vi "Prefilter_LP.vi"(8 "error in (no error)":errorcluster, 10 "low cutoff freq [Hz]":dbl=0.45, 11 "Waveforms In":waveform(dbl)[](array[waveform])) -> (0 "error out":errorcluster, 3 "Waveforms Out":waveform(dbl)[](array[waveform]))   [LabVIEW 2020, in "DSP_Filter.lvclass"]
uses:
  DSP_Filter.lvclass
  <vilib>/addons/Digital Filter Design/Process.llb/DFD Filtering (Wfm NChan).vi
  <vilib>/addons/Digital Filter Design/NI_DigFilterLicensed.lvlib
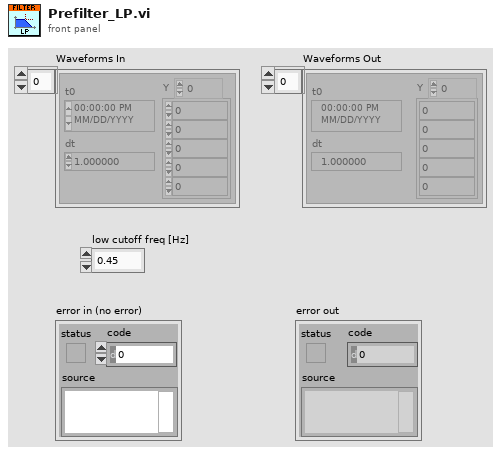
[diagram p1: front panel]
types:
  T1 = enum16{"Lowpass", "Highpass", "Bandpass", "Bandstop"}
  T2 = typedef "NI_DigFilterLicensed.lvlib/DFD Filter Obj.ctl" = cluster{"mSRate_Fs":dbl, "mSRate_Version":string, "mSRate_Comments":string, "mSRate_OrgCoef":T3, "mSRate_CurCoef":T3, "mSRate_Quantized?":bool, "mSRate_QCoef":T3, "mSRate_QSettings":T5[], "mSRate_Order":i32, "mSRate_Scaling":cluster{"mSRate_ScaleByPowerOf2?":bool, "mSRate_ScaleType":T7}}
  T3 = typedef "NI_DigFilterLicensed.lvlib/DFD Filter Coef.ctl" = cluster{"type":T4, "gain":dbl, "coef a (k)":dbl[], "coef b (v)":dbl[]}
  T4 = typedef "NI_DigFilterLicensed.lvlib/DFD Filter Structure Type Selector.ctl" = enum16{"Undefined", "FIR Direct Form", "FIR Direct Form Transposed", "FIR Symmetric", "FIR Antisymmetric", "IIR Direct Form I", "IIR Direct Form I Transposed", "IIR Direct Form II", "IIR Direct Form II Transposed", "IIR Cascaded Second Order Sections Form I", "IIR Cascaded Second Order Sections Form I Transposed", "IIR Cascaded Second Order Sections Form II", "IIR Cascaded Second Order Sections Form II Transposed", "Lattice Allpass (basic sections)", "Lattice Allpass (one multiplier sections)", "Lattice Allpass (normalized sections)", "Lattice AR (basic sections)", "Lattice AR (one multiplier sections)", "Lattice AR (normalized sections)", "Lattice MA (minimum phase)", "Lattice MA (maximum phase)", "Lattice ARMA (basic sections)", "Lattice ARMA (one multiplier sections)", "Lattice ARMA (normalized sections)"}
  T5 = typedef "NI_DigFilterLicensed.lvlib/dfd_Internal Quantization Settings.ctl" = cluster{"source":T6, "wl":i16, "iwl":i16, "overflow mode":enum16{"Saturation", "Wrap"}, "rounding mode":enum16{"Nearest", "Truncation"}, "signed?":bool}
  T6 = typedef "NI_DigFilterLicensed.lvlib/dfd_Internal Quantization Srcs.ctl" = u16
  T7 = typedef "NI_DigFilterLicensed.lvlib/DFD Coef Norm Type.ctl" = enum16{"No Norm", "Time Domain 1-Norm", "Time Domain 2-Norm", "Time Domain Inf-Norm"}
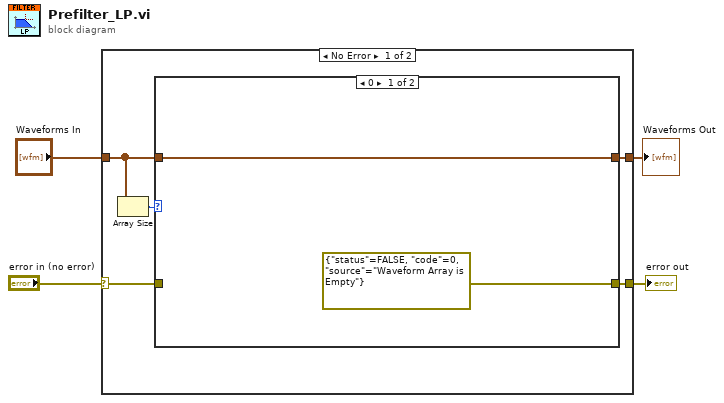
[diagram p0: block diagram]
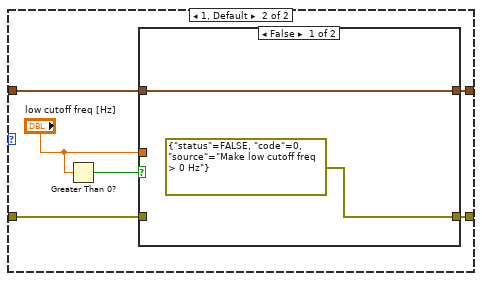
[diagram p2: hidden frame]
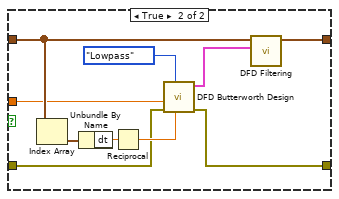
[diagram p3: hidden frame]
diagram:
  n1 = case shown="No Error" "error in (no error)" {
    selector: "error in (no error)" -> [w7 w30]
    tunnel: "Waveforms In" -> [w5 w31]
    tunnel: [w9 w31] -> w3
    tunnel: [w8 w30] -> w2
    frame No Error {
      n2 = Array Size(array=w5) -> (size(s)=w6:i32)
      n3 = case shown="0" w6 {
        tunnel: w5 -> [w10 w17]
        tunnel: [w10 w16] -> w9
        tunnel: [errorcluster {"status"=FALSE, "code"=0, "source"="Waveform Array is Empty"} ("error constant") w15] -> w8
        tunnel: w7 -> [_ w14]
        frame 0 {
        }
        frame 1, Default {
          n4 = Greater Than 0?(x="low cutoff freq [Hz]") -> (x > 0?=w12:bool)
          n5 = case shown="False" w12 {
            tunnel: w17 -> [w19 w27]
            tunnel: [w19 w26] -> w16
            tunnel: [errorcluster {"status"=FALSE, "code"=0, "source"="Make low cutoff freq > 0 Hz"} ("error constant") w22] -> w15
            tunnel: w14 -> [_ w21]
            tunnel: "low cutoff freq [Hz]" -> [_ w20]
            frame False {
            }
            frame True {
              n6 = Index Array(array=w27) -> (element=w28:waveform(dbl))  [unwired: 1 in]
              n7 = Unbundle By Name(w28) -> ("dt"=w29:dbl)
              n8 = Reciprocal(x=w29) -> (1/x=w25:dbl)
              n9 = call <vilib>:"DFD Butterworth Design.vi"("fs [Hz]"=w25, "filter type"=T1."Lowpass", "error in (no error)"=w21, "low cutoff freq [Hz]"=w20) -> ("error out"=w22:errorcluster, "filter out"=w24:T2)  [unwired: 6 in]
              n10 = call-poly <vilib>:"DFD Filtering.vi"("filter"=w24, "signal in"=w27) -> ("signal out"=w26:waveform(dbl)[])  [unwired: 8 in, 1 out]
            }
          }
        }
      }
    }
    frame Error {
    }
  }
  "Waveforms Out" <- w3
  "error out" <- w2
